vi "dash.vi"() -> ()   [LabVIEW 2022 SP3]
panel:
  out "Ignition State":bool
  in  "Ignition Safety":bool
  in  "Disconnect?":bool
  in  "Connect?":bool
  out "Switch 5":bool
  out "Switch 4":bool
  out "Switch 3":bool
  out "Switch 2":bool
  out "Switch 1":bool
  in  "Ignition":bool
  in  "Off 5":bool
  in  "Off 4":bool
  in  "Off 3":bool
  in  "Off 2":bool
  in  "Off 1":bool
  in  "On 5":bool
  in  "On 4":bool
  in  "On 3":bool
  in  "On 2":bool
  in  "On 1":bool
  out "Sensors":dbl[](array[numeric])
  out "Pressure Transducers":waveform(dbl)[](graph)
  out "Temperature":waveform(dbl)[](graph)
  out "Load Cells & Strain Gauges":waveform(dbl)[](graph)
  out "Console Message":string
  out "Raw JSON In":string
  in  "Address":string="192.168.1.114"
  in  "Port":i32=25005
  in  "Stop":bool
  # "LC0"
  # "LC 1"
  # "LC 2"
  # "LC 3"
  # "SG 0"
  # "SG 1"
  # "SG 3"
  # "SG 4"
  # "TC 2"
  # "TC 3"
  # "PT 0"
  # "PT 1"
  # "PT 2"
  # "PT 3"
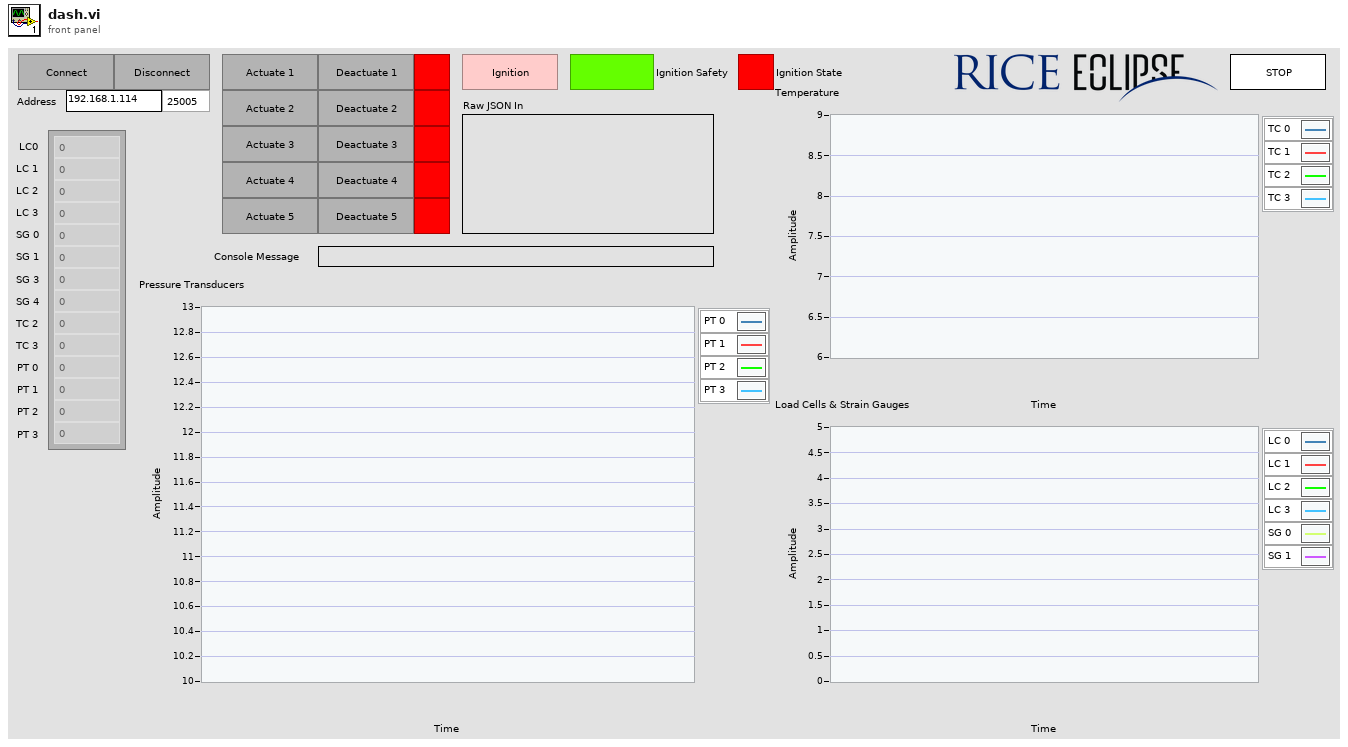
[diagram p1: front panel]
types:
  T1 = cluster{"command":string, "driver":i32, "value":i32}
  T2 = cluster{"states":i32[], "timestamp":string, "console":string, "sensors":dbl[]}
  T3 = cluster{"[0]":bool, "[1]":bool, "[2]":bool, "[3]":bool, "[4]":bool, "[5]":bool, "[6]":bool, "[7]":bool, "[8]":bool}
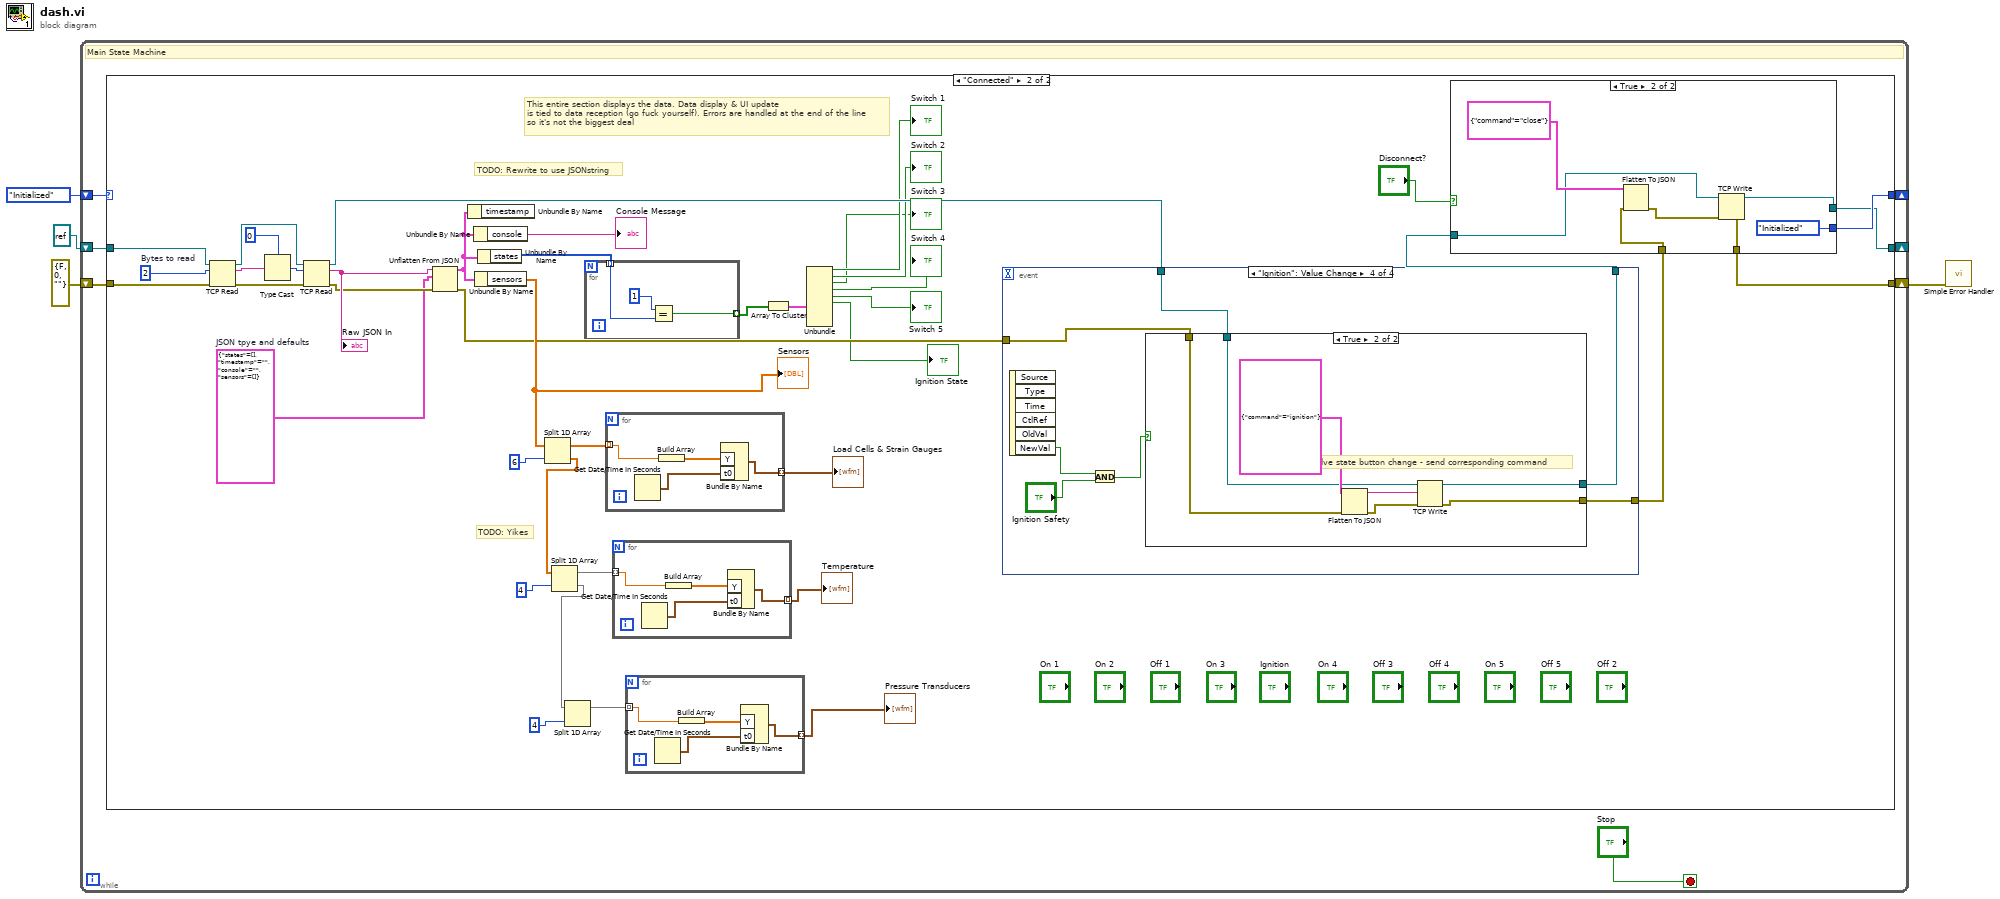
[diagram p0: block diagram]
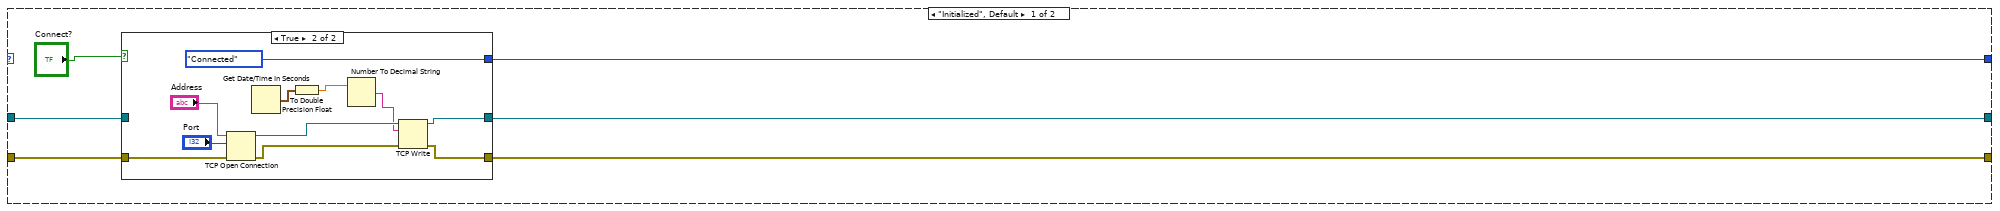
[diagram p2: hidden frame]
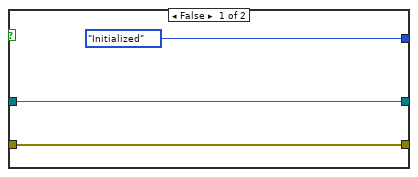
[diagram p3: hidden frame]
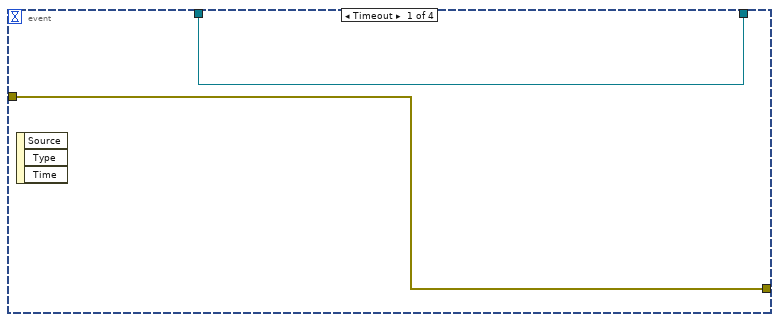
[diagram p4: hidden frame]
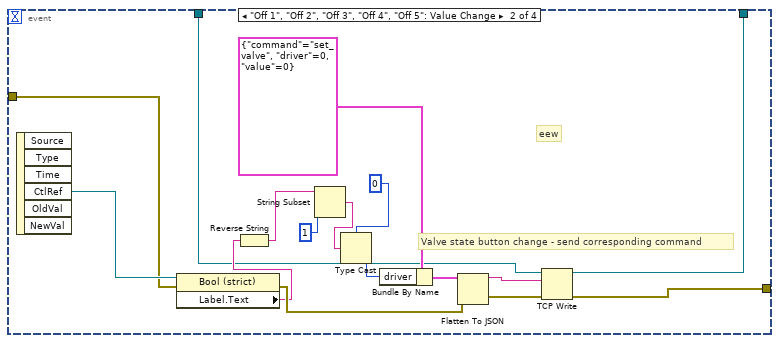
[diagram p5: hidden frame]
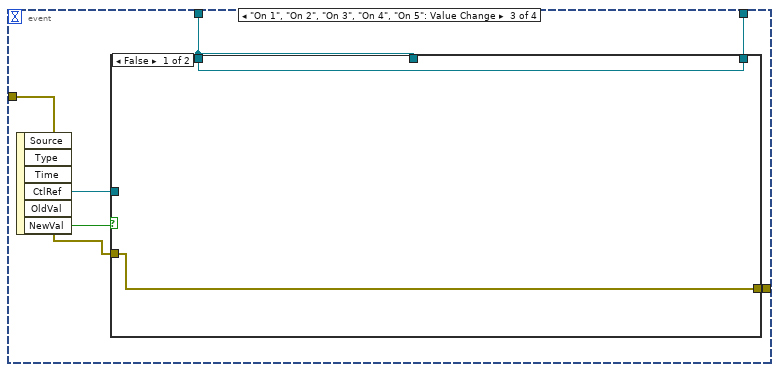
[diagram p6: hidden frame]
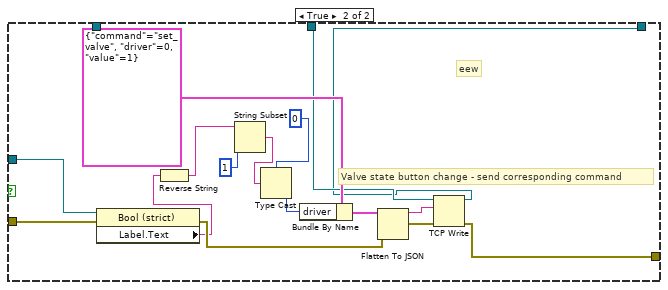
[diagram p7: hidden frame]
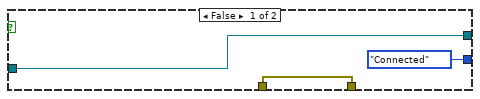
[diagram p9: hidden frame]
diagram:
  n1 = while {
    shift-right: [w10] -> _
    shift-left: enum16{"Initialized", "Connected"}."Initialized" -> [w11]
    shift-right: [w8] -> _
    shift-left: refnum<k5> refnum ("TCP Network Connection Refnum") -> [w5]
    shift-right: [w7] -> w1
    shift-left: errorcluster {"status"=FALSE, "code"=0, "source"=""} ("error constant") -> [w6]
    stop <- "Stop" stop-if-true
    # "Main State Machine"
    n2 = case shown="\"Connected\"" w11 {
      tunnel: [w17 w73] -> w10
      tunnel: [w16 w56] -> w8
      tunnel: [w15 w57] -> w7
      tunnel: w6 -> [w14 w66]
      tunnel: w5 -> [w13 w65]
      frame "Initialized", Default {
        n3 = case shown="True" "Connect?" {
          tunnel: [enum16{"Initialized", "Connected"}."Initialized" enum16{"Initialized", "Connected"}."Connected"] -> w17
          tunnel: [w19 w24] -> w16
          tunnel: [w18 w26] -> w15
          tunnel: w14 -> [w18 w29]
          tunnel: w13 -> [w19 _]
          frame False {
          }
          frame True {
            n4 = TCP Open Connection(address="Address", remote port or service name="Port", error in (no error)=w29) -> (connection ID=w25:refnum<k5>, error out=w27:errorcluster)  [unwired: 2 in]
            n5 = Get Date/Time In Seconds() -> (seconds since 1Jan1904=w23:timestamp)
            n6 = To Double Precision Float(number=w23) -> (double precision float=w22:dbl)
            n7 = Number To Decimal String(number=w22) -> (decimal integer string=w21:string)  [unwired: 1 in]
            n8 = TCP Write(connection ID=w25, data in=w21, error in (no error)=w27) -> (connection ID out=w24:refnum<k5>, error out=w26:errorcluster)  [unwired: 1 in, 1 out]
          }
        }
      }
      frame "Connected" {
        w61 = T2 {"states"=[], "timestamp"="", "console"="", "sensors"=[]}  # JSON tpye and defaults
        w72 = 2  # Bytes to read
        # "This entire section displays the data. Data display & UI update\nis tied to data reception (go fuck yourself). Errors are handled at the end of the line\nso it's not the biggest deal"
        # "TODO: Yikes"
        # "TODO: Rewrite to use JSONstring"
        n9 = TCP Read(connection ID=w65, bytes to read=w72, error in (no error)=w66) -> (connection ID out=w71:refnum<k5>, data out=w67:string, error out=w70:errorcluster)  [unwired: 2 in]
        n10 = Type Cast(type=u16 0, x=w67) -> (*(type *) &x=w68:u16)
        n11 = TCP Read(connection ID=w71, bytes to read=w68, error in (no error)=w70) -> (connection ID out=w43:refnum<k5>, data out=w63:string, error out=w62:errorcluster)  [unwired: 2 in]
        "Raw JSON In" <- w63
        n12 = Unflatten From JSON(JSON string=w63, type and defaults=w61, error in (no error)=w62) -> (value=w64:T2, error out=w45:errorcluster)  [unwired: 4 in]
        n13 = Unbundle By Name(w64) -> ()  [unwired: 1 out]
        n14 = Unbundle By Name(w64) -> ("console"=→"Console Message":string)
        n15 = Unbundle By Name(w64) -> ("sensors"=w46:dbl[])
        "Sensors" <- w46
        n16 = Unbundle By Name(w64) -> ("states"=w32:i32[])
        n17 = Split 1D Array(array=w46, index=6) -> (first subarray=w59:dbl[], second subarray=w52:dbl[])
        n18 = Split 1D Array(array=w52, index=4) -> (first subarray=w53:dbl[], second subarray=w48:dbl[])
        n19 = Split 1D Array(array=w48, index=4) -> (first subarray=w49:dbl[])  [unwired: 1 out]
        n20 = for {
          tunnel: w32 -> [w141] mode=indexing
          tunnel: [w140] -> w33 mode=indexing
          n21 = Equal?(x=1, y=w141) -> (x = y?=w140:bool)
        }
        n22 = for {
          tunnel: w59 -> [w145] mode=indexing
          tunnel: [w143] -> w55 mode=indexing
          n23 = Get Date/Time In Seconds() -> (seconds since 1Jan1904=w146:timestamp)
          n24 = Build Array(w145) -> (w144:dbl[])
          n25 = Bundle By Name("Y"=w144, "t0"=w146) -> (w143:waveform(dbl))  [unwired: 1 in]
        }
        "Load Cells & Strain Gauges" <- w55
        n26 = for {
          tunnel: w53 -> [w138] mode=indexing
          tunnel: [w136] -> w51 mode=indexing
          n27 = Get Date/Time In Seconds() -> (seconds since 1Jan1904=w139:timestamp)
          n28 = Build Array(w138) -> (w137:dbl[])
          n29 = Bundle By Name("Y"=w137, "t0"=w139) -> (w136:waveform(dbl))  [unwired: 1 in]
        }
        "Temperature" <- w51
        n30 = for {
          tunnel: w49 -> [w134] mode=indexing
          tunnel: [w132] -> w47 mode=indexing
          n31 = Get Date/Time In Seconds() -> (seconds since 1Jan1904=w135:timestamp)
          n32 = Build Array(w134) -> (w133:dbl[])
          n33 = Bundle By Name("Y"=w133, "t0"=w135) -> (w132:waveform(dbl))  [unwired: 1 in]
        }
        "Pressure Transducers" <- w47
        n34 = Array To Cluster(array=w33) -> (cluster=w41:T3)
        n35 = Unbundle(w41) -> ("[0]"=→"Switch 1":bool, "[1]"=→"Switch 2":bool, "[2]"=→"Switch 3":bool, "[3]"=→"Switch 4":bool, "[4]"=→"Switch 5":bool, "[5]"=→"Ignition State":bool)  [unwired: 3 out]
        n36 = event shown="[3] \"Ignition\": Value Change" {
          selector: _ -> [_ _ _ _]
          dyn-events: _ -> [_ _ _ _]
          timeout: _ -> [_ _ _ _]
          tunnel: w45 -> [w75 w79 w95 w122]
          tunnel: [w75 w78 w94 w121] -> w44
          tunnel: w43 -> [w74 w77 w92 w120]
          tunnel: [w74 w76 w93 w119] -> w42
          event Timeout {
            n37 = event-data() -> ()  [unwired: 1 in, 3 out]
          }
          event "Off 1", "Off 2", "Off 3", "Off 4", "Off 5": Value Change {
            # "eew"
            # "Valve state button change - send corresponding command"
            n38 = event-data() -> ("CtlRef"=w80:refnum<vi>)  [unwired: 1 in, 5 out]
            n39 = property class="Bool (strict)"(reference=w80, error in=w79) -> (error out=w88:errorcluster, "Label.Text"=w86:string)  [unwired: 1 out]
            n40 = Reverse String(1:w86) -> (0:w85:string)
            n41 = String Subset(string=w85, length (rest)=1) -> (substring=w83:string)  [unwired: 1 in]
            n42 = Type Cast(type=0, x=w83) -> (*(type *) &x=w81:i32)
            n43 = Bundle By Name(cluster=T1 {"command"="set_valve", "driver"=0, "value"=0}, "driver"=w81) -> (w90:T1)
            n44 = Flatten To JSON(anything=w90, error in (no error)=w88) -> (JSON string=w89:string, 11:w87:errorcluster)  [unwired: 1 in]
            n45 = TCP Write(connection ID=w77, data in=w89, error in (no error)=w87) -> (connection ID out=w76:refnum<k5>, error out=w78:errorcluster)  [unwired: 1 in, 1 out]
          }
          event "On 1", "On 2", "On 3", "On 4", "On 5": Value Change {
            n46 = event-data() -> ("CtlRef"=w96:refnum<vi>, "NewVal"=w97:bool)  [unwired: 1 in, 4 out]
            n47 = case shown="False" w97 {
              tunnel: w96 -> [_ w112]
              tunnel: w95 -> [w99 w109]
              tunnel: [w99 w102] -> w94
              tunnel: w92 -> [_ w101]
              tunnel: [w98 w100] -> w93
              tunnel: w92 -> [w98 _]
              frame False {
              }
              frame True {
                # "eew"
                # "Valve state button change - send corresponding command"
                n48 = property class="Bool (strict)"(reference=w112, error in=w109) -> (error out=w111:errorcluster, "Label.Text"=w108:string)  [unwired: 1 out]
                n49 = Reverse String(1:w108) -> (0:w107:string)
                n50 = String Subset(string=w107, length (rest)=1) -> (substring=w105:string)  [unwired: 1 in]
                n51 = Type Cast(type=0, x=w105) -> (*(type *) &x=w103:i32)
                n52 = Bundle By Name(cluster=T1 {"command"="set_valve", "driver"=0, "value"=1}, "driver"=w103) -> (w114:T1)
                n53 = Flatten To JSON(anything=w114, error in (no error)=w111) -> (JSON string=w113:string, 11:w110:errorcluster)  [unwired: 1 in]
                n54 = TCP Write(connection ID=w101, data in=w113, error in (no error)=w110) -> (connection ID out=w100:refnum<k5>, error out=w102:errorcluster)  [unwired: 1 in, 1 out]
              }
            }
          }
          event "Ignition": Value Change {
            n55 = event-data() -> ("NewVal"=w117:bool)  [unwired: 1 in, 5 out]
            n56 = And(x=w117, y="Ignition Safety") -> (x .and. y?=w116:bool)
            n57 = case shown="True" w116 {
              tunnel: w122 -> [w124 w130]
              tunnel: [w124 w127] -> w121
              tunnel: w120 -> [w123 w129]
              tunnel: [w123 w126] -> w119
              frame False {
              }
              frame True {
                # "Valve state button change - send corresponding command"
                n58 = Flatten To JSON(anything=cluster{"command":string} {"command"="ignition"}, error in (no error)=w130) -> (JSON string=w125:string, 11:w128:errorcluster)  [unwired: 1 in]
                n59 = TCP Write(connection ID=w129, data in=w125, error in (no error)=w128) -> (connection ID out=w126:refnum<k5>, error out=w127:errorcluster)  [unwired: 1 in, 1 out]
              }
            }
          }
        }
        n60 = case shown="True" "Disconnect?" {
          tunnel: [enum16{"Initialized", "Connected"}."Connected" enum16{"Initialized", "Connected"}."Initialized"] -> w73
          tunnel: w42 -> [w148 w150]
          tunnel: [w147 w155] -> w57
          tunnel: [w148 w154] -> w56
          tunnel: w44 -> [w147 w152]
          frame False {
          }
          frame True {
            n61 = Flatten To JSON(anything=cluster{"command":string} {"command"="close"}, error in (no error)=w152) -> (11:w153:errorcluster)  [unwired: 1 in, 1 out]
            n62 = TCP Write(connection ID=w150, error in (no error)=w153) -> (connection ID out=w154:refnum<k5>, error out=w155:errorcluster)  [unwired: 2 in, 1 out]
          }
        }
      }
    }
  }
  n63 = call <vilib>:"Simple Error Handler.vi"("error in (no error)"=w1) -> ()  [unwired: 4 in, 5 out]
